vi "Get only Top VI elements.vi"(1 "Ref. array in":refnum<vi>[](array[refnum]), 2 "VI ref.":refnum<vi>) -> (0 "Ref. array out":refnum<vi>[](array[refnum]))   [LabVIEW 2014]
doc: "Return objects reference numbers which are owned directly by VI, so if there is nested WhileLoop, or any other object its refnum would be erased."
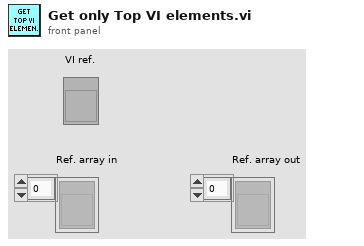
[diagram p1: front panel]
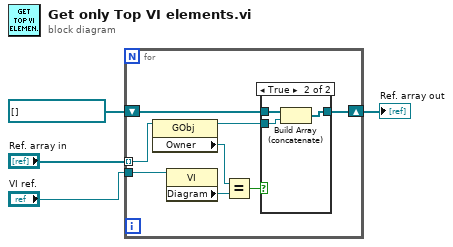
[diagram p0: block diagram]
diagram:
  n1 = for {
    tunnel: "Ref. array in" -> [w12] mode=indexing
    shift-right: [w8] -> w4
    shift-left: refnum<vi>[] [] -> [w7]
    tunnel: "VI ref." -> [w5]
    n2 = property class="GObj"(reference=w12) -> (reference out=w6:refnum<vi>, "Owner"=w11:refnum<vi>)  [unwired: 1 in, 1 out]
    n3 = property class="VI"(reference=w5) -> ("Diagram"=w10:refnum<vi>)  [unwired: 1 in, 2 out]
    n4 = Equal?(x=w11, y=w10) -> (x = y?=w9:bool)
    n5 = case shown="True" w9 {
      tunnel: [w13 w16] -> w8
      tunnel: w7 -> [w13 w15]
      tunnel: w6 -> [_ w14]
      frame False {
      }
      frame True {
        n6 = Build Array (concatenate)(w15, w14) -> (w16:refnum<vi>[])
      }
    }
  }
  "Ref. array out" <- w4
